vi "Devcon.Remove Devices.vi"(8 "error in (no error)":errorcluster, 9 "State(Present(F), All(T))":bool, 10 "DeviceID":string="USB\\VID_28DE&PID_2300&MI_02\\9&35BD5232&0&0002", 11 "DevconEXE":path=path "C:/Program Files (x86)/Windows Kits/10/Tools/x64/devcon") -> (0 "error out":errorcluster, 1 "FailCnt":i32, 2 "RemoveCnt":i32, 3 "Success":bool, 4 "Device List":string[][](array[string]))   [LabVIEW 2018]
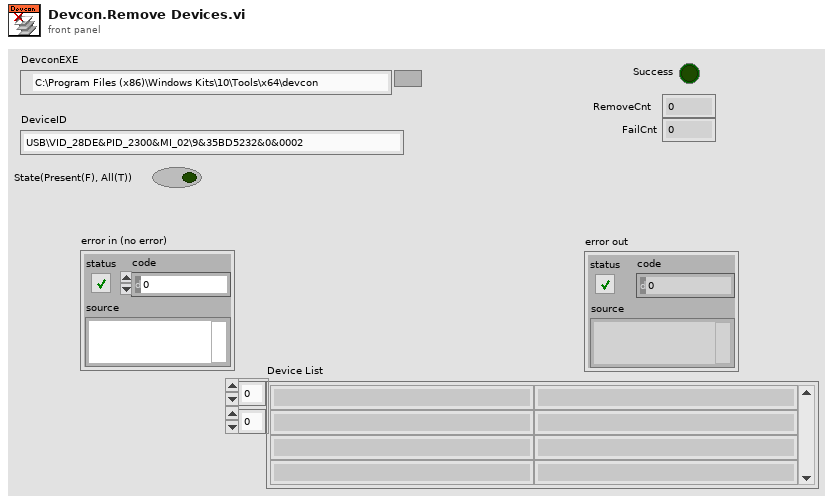
[diagram p1: front panel]
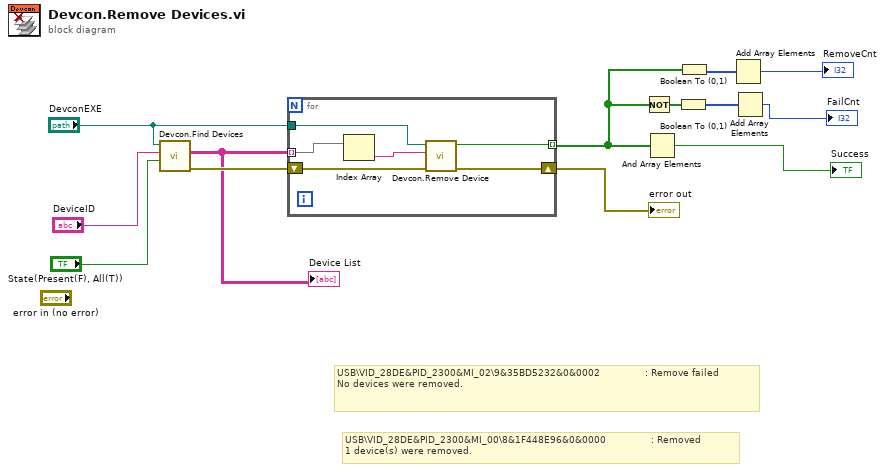
[diagram p0: block diagram]
diagram:
  # "USB\\VID_28DE&PID_2300&MI_00\\8&1F448E96&0&0000               : Removed\n1 device(s) were removed."
  # "USB\\VID_28DE&PID_2300&MI_02\\9&35BD5232&0&0002               : Remove failed\nNo devices were removed."
  n1 = call "Devcon.Find Devices.vi"("State(Present(F), All(T))"="State(Present(F), All(T))", "DeviceID"="DeviceID", "DevconEXE"="DevconEXE") -> ("error out"=w11:errorcluster, "Device List"=w3:string[][])  [unwired: 4 in, 3 out]
  "Device List" <- w3
  n2 = for {
    tunnel: w3 -> [w18] mode=indexing
    tunnel: "DevconEXE" -> [w19]
    shift-right: [w15] -> w10
    shift-left: w11 -> [w16]
    tunnel: [w14] -> w8 mode=indexing
    n3 = Index Array(array=w18) -> (element=w17:string)  [unwired: 1 in]
    n4 = call "Devcon.Remove Device.vi"("error in (no error)"=w16, "DeviceID"=w17, "DevconEXE"=w19) -> ("error out"=w15:errorcluster, "Success"=w14:bool)  [unwired: 5 in, 2 out]
  }
  "error out" <- w10
  n5 = Not(x=w8) -> (.not. x?=w9:bool[])
  n6 = And Array Elements(Boolean array=w8) -> (logical AND=→"Success":bool)
  n7 = Boolean To (0,1)(Boolean=w9) -> (0, 1=w5:i16[])
  n8 = Boolean To (0,1)(Boolean=w8) -> (0, 1=w7:i16[])
  n9 = Add Array Elements(numeric array=w7) -> (sum=→"RemoveCnt":i16)
  n10 = Add Array Elements(numeric array=w5) -> (sum=→"FailCnt":i16)
